vi "Read Parameters.vi"(8 "error in (no error)":errorcluster, 11 "Drive by Power in":refnum<class "Drive by Power.lvclass">) -> (0 "error out":errorcluster, 1 "Parameters String":string, 2 "Parameters":T1 {"Right Power" min=-1.0 max=1.0; "Left Power" min=-1.0 max=1.0}, 3 "Drive by Power out":refnum<class "Drive by Power.lvclass">)   [LabVIEW 2014, in "Forward Drive.lvlib" / "Drive by Power.lvclass"]
uses:
  Drive by Power.lvclass
  Parameters.ctl
  Drive by Power.lvclass/Drive by Power.ctl
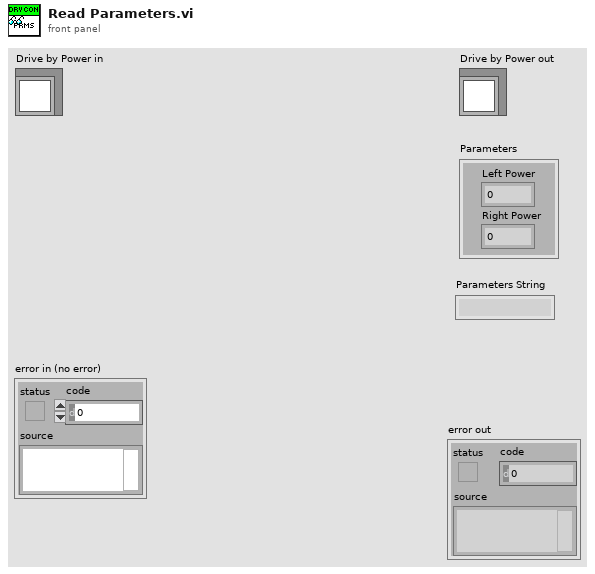
[diagram p1: front panel]
types:
  T1 = typedef "Forward Drive.lvlib/Drive by Power.lvclass/Parameters.ctl" = cluster{"Left Power":dbl, "Right Power ":dbl}
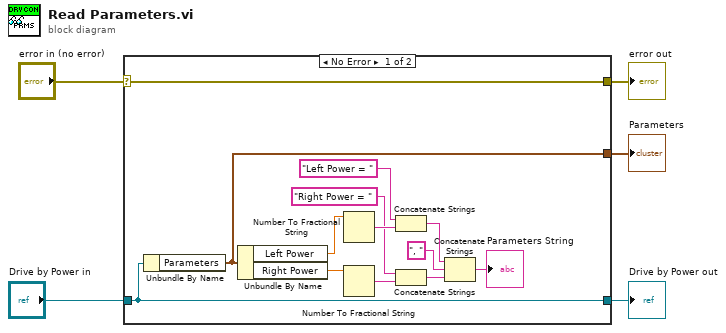
[diagram p0: block diagram]
diagram:
  n1 = case shown="No Error" "error in (no error)" {
    selector: "error in (no error)" -> [w18 w19]
    tunnel: [w18 w19] -> w4
    tunnel: [w17 w20] -> w2
    tunnel: "Drive by Power in" -> [w17 w20]
    tunnel: [w16 _] -> w1
    frame No Error {
      n2 = Unbundle By Name(w17) -> ("Parameters"=w16:T1)
      n3 = Unbundle By Name(w16) -> ("Left Power"=w15:dbl, "Right Power"=w7:dbl)
      n4 = Number To Fractional String(number=w15) -> (F-format string=w11:string)  [unwired: 3 in]
      n5 = Number To Fractional String(number=w7) -> (F-format string=w9:string)  [unwired: 3 in]
      n6 = Concatenate Strings("Left Power = " ("string"), w11) -> (w14:string)
      n7 = Concatenate Strings("Right Power = " ("string"), w9) -> (w12:string)
      n8 = Concatenate Strings(w14, ", " ("string"), w12) -> (→"Parameters String":string)
    }
    frame Error {
    }
  }
  "error out" <- w4
  "Drive by Power out" <- w2
  "Parameters" <- w1
